vi "solar_app Window Resize.vi"(8 "error in (no error)":errorcluster, 10 "New FP.WinBounds":T1, 11 "VI Refnum":refnum<vi>) -> (0 "error out":errorcluster, 2 "Resolved FP.WinBounds":T1, 3 "dup VI Refnum":refnum<vi>)   [LabVIEW 2018]
doc: "This resizes a front panel window."
uses:
  <vilib>/Utility/miscctls.llb/LVRectTypeDef.ctl
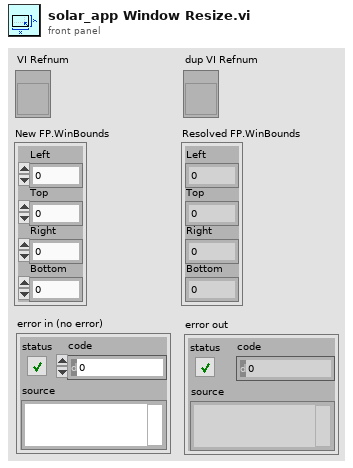
[diagram p1: front panel]
types:
  T1 = typedef "LVRectTypeDef.ctl" = cluster{"Left":i16, "Top":i16, "Right":i16, "Bottom":i16}
  T2 = typedef "LVPointTypeDef.ctl" = cluster{"Horizontal":i16, "Vertical":i16}
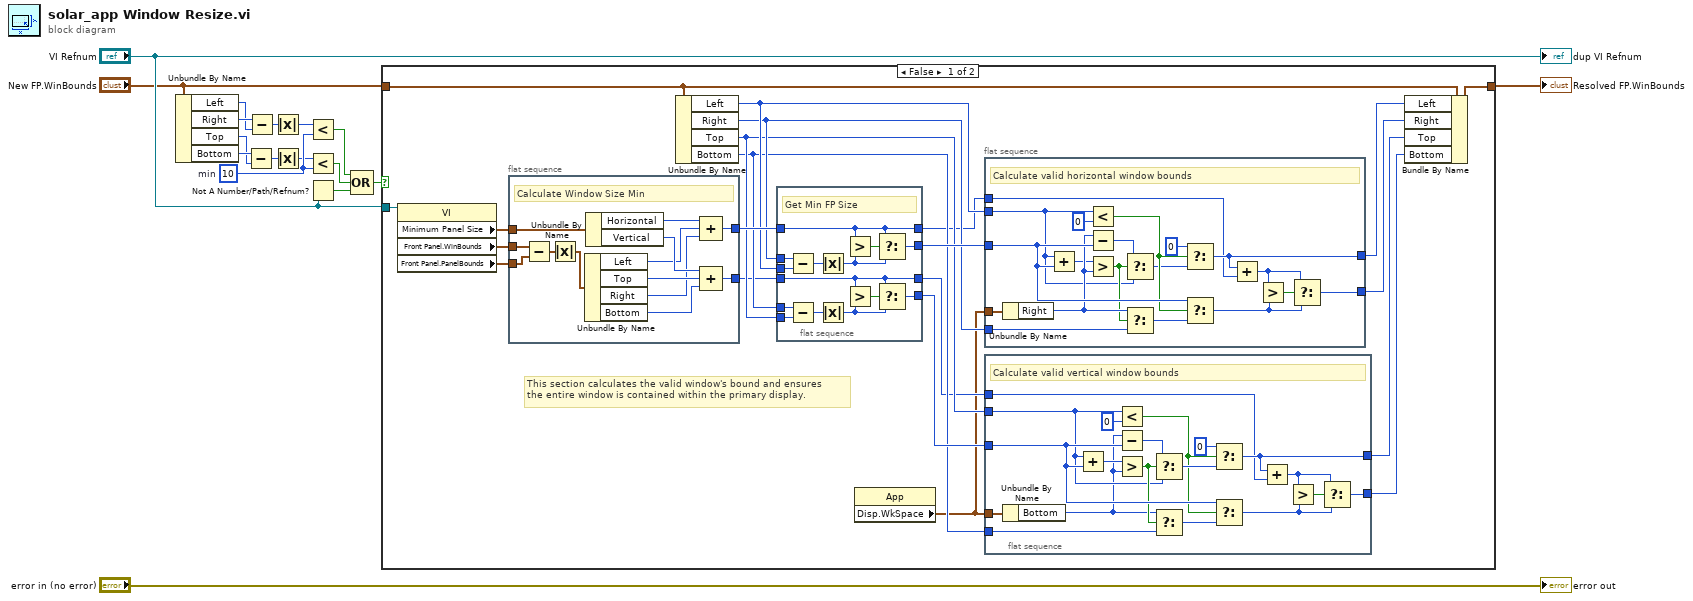
[diagram p0: block diagram]
diagram:
  w7 = i16 10  # min
  n1 = Unbundle By Name("New FP.WinBounds") -> ("Left"=w12:i16, "Right"=w13:i16, "Top"=w10:i16, "Bottom"=w11:i16)
  n2 = Subtract(x=w11, y=w10) -> (x-y=w8:i16)
  n3 = Subtract(x=w13, y=w12) -> (x-y=w9:i16)
  n4 = Absolute Value(x=w9) -> (abs(x)=w2:i16)
  n5 = Absolute Value(x=w8) -> (abs(x)=w1:i16)
  n6 = Less?(x=w2, y=w7) -> (x < y?=w6:bool)
  n7 = Less?(x=w1, y=w7) -> (x < y?=w5:bool)
  n8 = Not A Number/Path/Refnum?(number/path/refnum="VI Refnum") -> (NaN/Path/Refnum?=w4:bool)
  n9 = Compound Arithmetic op=OR(w6, w5, w4) -> (w3:bool)
  n10 = case "Invalid Refnum?" shown="False" w3 {
    tunnel: "New FP.WinBounds" -> [w38 w104]
    tunnel: [w37 w104] -> w17
    tunnel: "VI Refnum" -> [w33 _]
    frame False {
      # "This section calculates the valid window's bound and ensures\nthe entire window is contained within the primary display."
      n11 = property class="VI"(reference=w33) -> ("Minimum Panel Size"=w36:T2, "Front Panel.WinBounds"=w35:T1, "Front Panel.PanelBounds"=w34:T1)  [unwired: 1 in, 2 out]
      n12 = flat-sequence {
        tunnel: [w103] -> w32
        tunnel: w36 -> [w96]
        tunnel: [w95] -> w21
        tunnel: w35 -> [w93]
        tunnel: w34 -> [w92]
        frame #0 {
          # "Calculate Window Size Min"
          n13 = Subtract(x=w93, y=w92) -> (x-y=w94:T1)
          n14 = Absolute Value(x=w94) -> (abs(x)=w91:T1)
          n15 = Unbundle By Name(w91) -> ("Left"=w97:i16, "Top"=w101:i16, "Right"=w99:i16, "Bottom"=w102:i16)
          n16 = Unbundle By Name(w96) -> ("Horizontal"=w98:i16, "Vertical"=w100:i16)
          n17 = Compound Arithmetic op=ADD(w98, w97, w99) -> (w103:i16)
          n18 = Compound Arithmetic op=ADD(w100, w101, w102) -> (w95:i16)
        }
      }
      n19 = Unbundle By Name(w38) -> ("Left"=w29:i16, "Right"=w28:i16, "Top"=w27:i16, "Bottom"=w26:i16)
      n20 = flat-sequence {
        tunnel: w32 -> [w77]
        tunnel: [w90] -> w31
        tunnel: [w89] -> w30
        tunnel: w29 -> [w82]
        tunnel: w28 -> [w81]
        tunnel: w27 -> [w80]
        tunnel: w26 -> [w79]
        tunnel: w21 -> [w78]
        tunnel: [w78] -> w20
        tunnel: [w77] -> w19
        frame #0 {
          # "Get Min FP Size"
          n21 = Subtract(x=w81, y=w82) -> (x-y=w83:i16)
          n22 = Subtract(x=w79, y=w80) -> (x-y=w84:i16)
          n23 = Absolute Value(x=w83) -> (abs(x)=w86:i16)
          n24 = Absolute Value(x=w84) -> (abs(x)=w88:i16)
          n25 = Greater?(x=w77, y=w86) -> (0:w85:bool)
          n26 = Greater?(x=w78, y=w88) -> (0:w87:bool)
          n27 = Select(t=w77, s=w85, f=w86) -> (s? t:f=w89:i16)
          n28 = Select(t=w78, s=w87, f=w88) -> (s? t:f=w90:i16)
        }
      }
      n29 = property class="App"() -> ("Disp.WkSpace"=w18:T1)  [unwired: 2 in, 2 out]
      n30 = flat-sequence {
        tunnel: w30 -> [w54]
        tunnel: w29 -> [w44]
        tunnel: w28 -> [w43]
        tunnel: [w42] -> w25
        tunnel: [w41] -> w24
        tunnel: w19 -> [w40]
        tunnel: w18 -> [w39]
        frame #0 {
          # "Calculate valid horizontal window bounds"
          n31 = Unbundle By Name(w39) -> ("Right"=w53:i16)
          n32 = Add(x=w44, y=w54) -> (x+y=w45:i16)
          n33 = Less?(x=w44, y=i16 0) -> (x < y?=w51:bool)
          n34 = Subtract(x=w53, y=w54) -> (x-y=w47:i16)
          n35 = Greater?(x=w45, y=w53) -> (0:w48:bool)
          n36 = Select(t=w47, s=w48, f=w44) -> (s? t:f=w49:i16)
          n37 = Select(t=w53, s=w48, f=w43) -> (s? t:f=w50:i16)
          n38 = Select(t=i16 0, s=w51, f=w49) -> (s? t:f=w42:i16)
          n39 = Select(t=w54, s=w51, f=w50) -> (s? t:f=w57:i16)
          n40 = Add(x=w42, y=w40) -> (x+y=w56:i16)
          n41 = Greater?(x=w56, y=w57) -> (0:w55:bool)
          n42 = Select(t=w56, s=w55, f=w57) -> (s? t:f=w41:i16)
        }
      }
      n43 = flat-sequence {
        tunnel: w31 -> [w73]
        tunnel: w27 -> [w64]
        tunnel: w26 -> [w63]
        tunnel: [w62] -> w23
        tunnel: [w61] -> w22
        tunnel: w20 -> [w60]
        tunnel: w18 -> [w59]
        frame #0 {
          # "Calculate valid vertical window bounds"
          n44 = Unbundle By Name(w59) -> ("Bottom"=w58:i16)
          n45 = Add(x=w64, y=w73) -> (x+y=w72:i16)
          n46 = Less?(x=w64, y=i16 0) -> (x < y?=w66:bool)
          n47 = Subtract(x=w58, y=w73) -> (x-y=w70:i16)
          n48 = Greater?(x=w72, y=w58) -> (0:w69:bool)
          n49 = Select(t=w70, s=w69, f=w64) -> (s? t:f=w68:i16)
          n50 = Select(t=w58, s=w69, f=w63) -> (s? t:f=w67:i16)
          n51 = Select(t=i16 0, s=w66, f=w68) -> (s? t:f=w62:i16)
          n52 = Select(t=w73, s=w66, f=w67) -> (s? t:f=w76:i16)
          n53 = Add(x=w62, y=w60) -> (x+y=w74:i16)
          n54 = Greater?(x=w74, y=w76) -> (0:w75:bool)
          n55 = Select(t=w74, s=w75, f=w76) -> (s? t:f=w61:i16)
        }
      }
      n56 = Bundle By Name(cluster=w38, "Left"=w25, "Right"=w24, "Top"=w23, "Bottom"=w22) -> (w37:T1)
    }
    frame True {
      # "Invalid Window Size"
    }
  }
  "Resolved FP.WinBounds" <- w17
  "dup VI Refnum" <- "VI Refnum"
  "error out" <- "error in (no error)"
